vi "Create ToolStripProgressBar by Name and width.vi"(8 "error in (no error)":errorcluster caption="错误输入（无错误）", 10 "Width":i32, 11 "name":string) -> (0 "error out":errorcluster caption="错误输出", 2 "Item":refnum<k24>, 3 "ToolStripProgressBar 输出":refnum<class "ToolStripProgressBar.lvclass"> caption="DNL_LabVIEW Object out")   [LabVIEW 2013, in "ToolStripProgressBar.lvclass"]
uses:
  ToolStripProgressBar.lvclass
  System.Windows.Forms
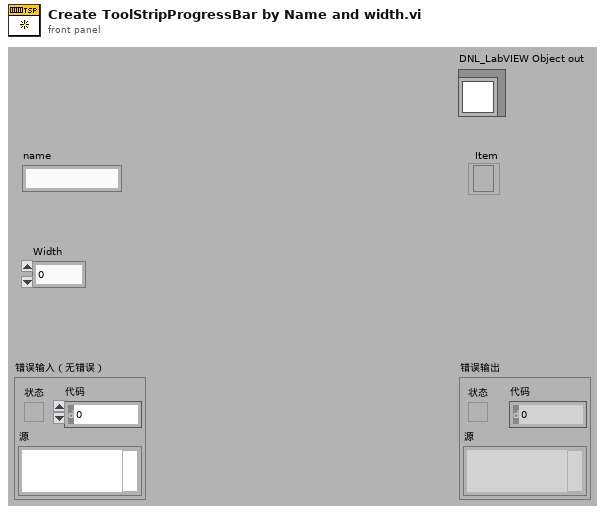
[diagram p1: front panel]
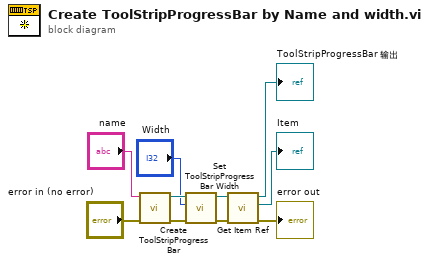
[diagram p0: block diagram]
diagram:
  n1 = call "Create ToolStripProgressBar.vi"("error in (no error)"="error in (no error)", "name"="name") -> ("error out"=w8:errorcluster, "ToolStripProgressBar 输出"=w10:refnum<class "ToolStripProgressBar.lvclass">)  [unwired: 8 in]
  n2 = call "Set ToolStripProgressBar Width.vi"("error in (no error)"=w8, "Width"="Width", "ToolStripProgressBar 输入"=w10) -> ("error out"=w4:errorcluster, "ToolStripProgressBar 输出"=w5:refnum<class "ToolStripProgressBar.lvclass">)  [unwired: 7 in]
  n3 = call "Get Item Ref.vi"("error in (no error)"=w4, "ToolStripProgressBar 输入"=w5) -> ("error out"=→"error out":errorcluster, "Item"=→"Item":refnum<k24>, "ToolStripProgressBar 输出"=→"ToolStripProgressBar 输出":refnum<class "ToolStripProgressBar.lvclass">)  [unwired: 7 in]
